vi "Channel Array to Channel List String.vi"(10 "Channel Array":T1(array[cluster])) -> (2 "Channel List String":string)   [LabVIEW 2018, in "Keithley 3706.lvlib"]
uses:
  <instrlib>/Keithley 3706/Keithley 3706.lvlib
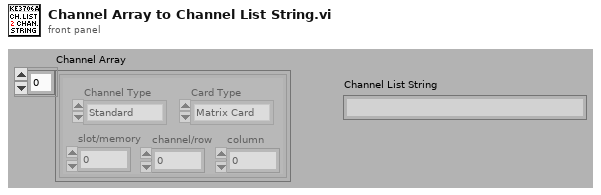
[diagram p1: front panel]
types:
  T1 = cluster{"slot/memory":i32, "channel/row":i32, "column":i32, "Channel Type":enum16{"Standard"}, "Card Type":enum16{"Matrix Card", "Multiplexer Card"}}[]
  T2 = cluster{"slot/memory":i32, "channel/row":i32, "column":i32, "Channel Type":enum16{"Standard"}, "Card Type":enum16{"Matrix Card", "Multiplexer Card"}}
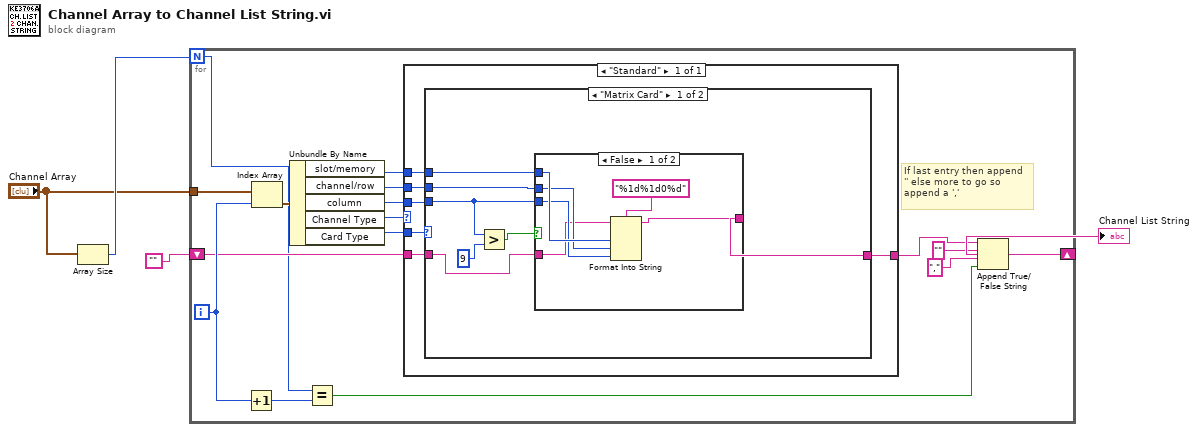
[diagram p0: block diagram]
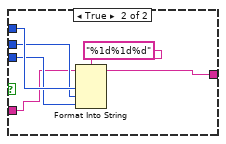
[diagram p2: hidden frame]
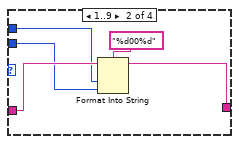
[diagram p4: hidden frame]
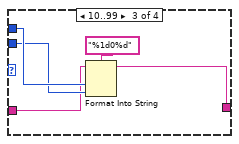
[diagram p5: hidden frame]
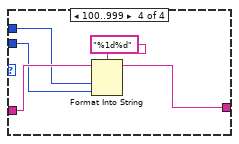
[diagram p6: hidden frame]
diagram:
  n1 = Array Size(array="Channel Array") -> (size(s)=w3:i32)
  n2 = for {
    N: w3 -> [w5]
    tunnel: "Channel Array" -> [w20]
    shift-right: [w7] -> w4
    shift-left: "" -> [w16]
    i -> [w19]
    # "If last entry then append\n'' else more to go so\nappend a ','"
    n3 = Increment(x=w19) -> (x+1=w6:i32)
    n4 = Index Array(array=w20, index=w19) -> (element=w18:T2)
    n5 = Unbundle By Name(w18) -> ("slot/memory"=w15:i32, "channel/row"=w13:i32, "column"=w12:i32, "Channel Type"=w17:enum16{"Standard"}, "Card Type"=w14:enum16{"Matrix Card", "Multiplexer Card"})
    n6 = Equal?(x=w5, y=w6) -> (x = y?=w10:bool)
    n7 = case shown="\"Standard\"" w17 {
      tunnel: w16 -> [w25]
      tunnel: w15 -> [w24]
      tunnel: [w21] -> w11
      tunnel: w14 -> [w26]
      tunnel: w13 -> [w23]
      tunnel: w12 -> [w22]
      frame "Standard" {
        n8 = case shown="\"Matrix Card\"" w26 {
          tunnel: w25 -> [w27 w47]
          tunnel: w24 -> [w31 w49]
          tunnel: w23 -> [w30 w48]
          tunnel: [w28 w46] -> w21
          tunnel: w22 -> [w29 _]
          frame "Matrix Card" {
            n9 = Greater?(x=w29, y=9) -> (0:w32:bool)
            n10 = case shown="False" w32 {
              tunnel: w31 -> [w39 w45]
              tunnel: w30 -> [w38 w44]
              tunnel: w29 -> [w37 w43]
              tunnel: [w34 w41] -> w28
              tunnel: w27 -> [w36 w40]
              frame False {
                n11 = Format Into String(format string="%1d%1d0%d", initial string=w36, w39, w38, w37) -> (resulting string=w34:string)  [unwired: 1 in, 1 out]
              }
              frame True {
                n12 = Format Into String(format string="%1d%1d%d", initial string=w40, w45, w44, w43) -> (resulting string=w41:string)  [unwired: 1 in, 1 out]
              }
            }
          }
          frame "Multiplexer Card" {
            n13 = case shown="0, Default" w48 {
              tunnel: w49 -> [_ w54 w60 w64]
              tunnel: w48 -> [_ w53 w59 w63]
              tunnel: w47 -> [w50 w55 w58 w65]
              tunnel: [w50 w51 w57 w61] -> w46
              frame 0, Default {
              }
              frame 1..9 {
                n14 = Format Into String(format string="%d00%d", initial string=w55, w54, w53) -> (resulting string=w51:string)  [unwired: 1 in, 1 out]
              }
              frame 10..99 {
                n15 = Format Into String(format string="%1d0%d", initial string=w58, w60, w59) -> (resulting string=w57:string)  [unwired: 1 in, 1 out]
              }
              frame 100..999 {
                n16 = Format Into String(format string="%1d%d", initial string=w65, w64, w63) -> (resulting string=w61:string)  [unwired: 1 in, 1 out]
              }
            }
          }
        }
      }
    }
    n17 = Append True/False String(1:w10, 2:",", 3:"", 4:w11) -> (0:w7:string)
  }
  "Channel List String" <- w4
